vi "GOOP_VI_Item_OnPopupMenu.vi"(11 "Object":u64) -> ()   [LabVIEW 2012]
uses:
  <resource>/Framework/Providers/API/mxLvMenuItem.ctl
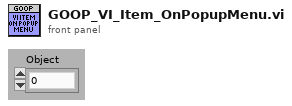
[diagram p1: front panel]
types:
  T1 = typedef "mxLvMenuItem.ctl" = cluster{"Menu Name":string, "Description":string, "Icon File Name":path, "Menu Tag":string, "Enabled":bool, "Checked":bool, "Separator":bool, "Batchable":bool, "Weight":i32, "Batch Mode (Ignored if Not Batchable)":enum32{"Show If All Items Support Command", "Show If Any Items Support Command"}, "Menu Location":enum32{"<None>", "Project", "Project / Build Specifications", "Tools", "Tools / Source Control", "Tools / Real-Time Module", "Help"}, "Exclude From Getting Started Window Menu":bool}
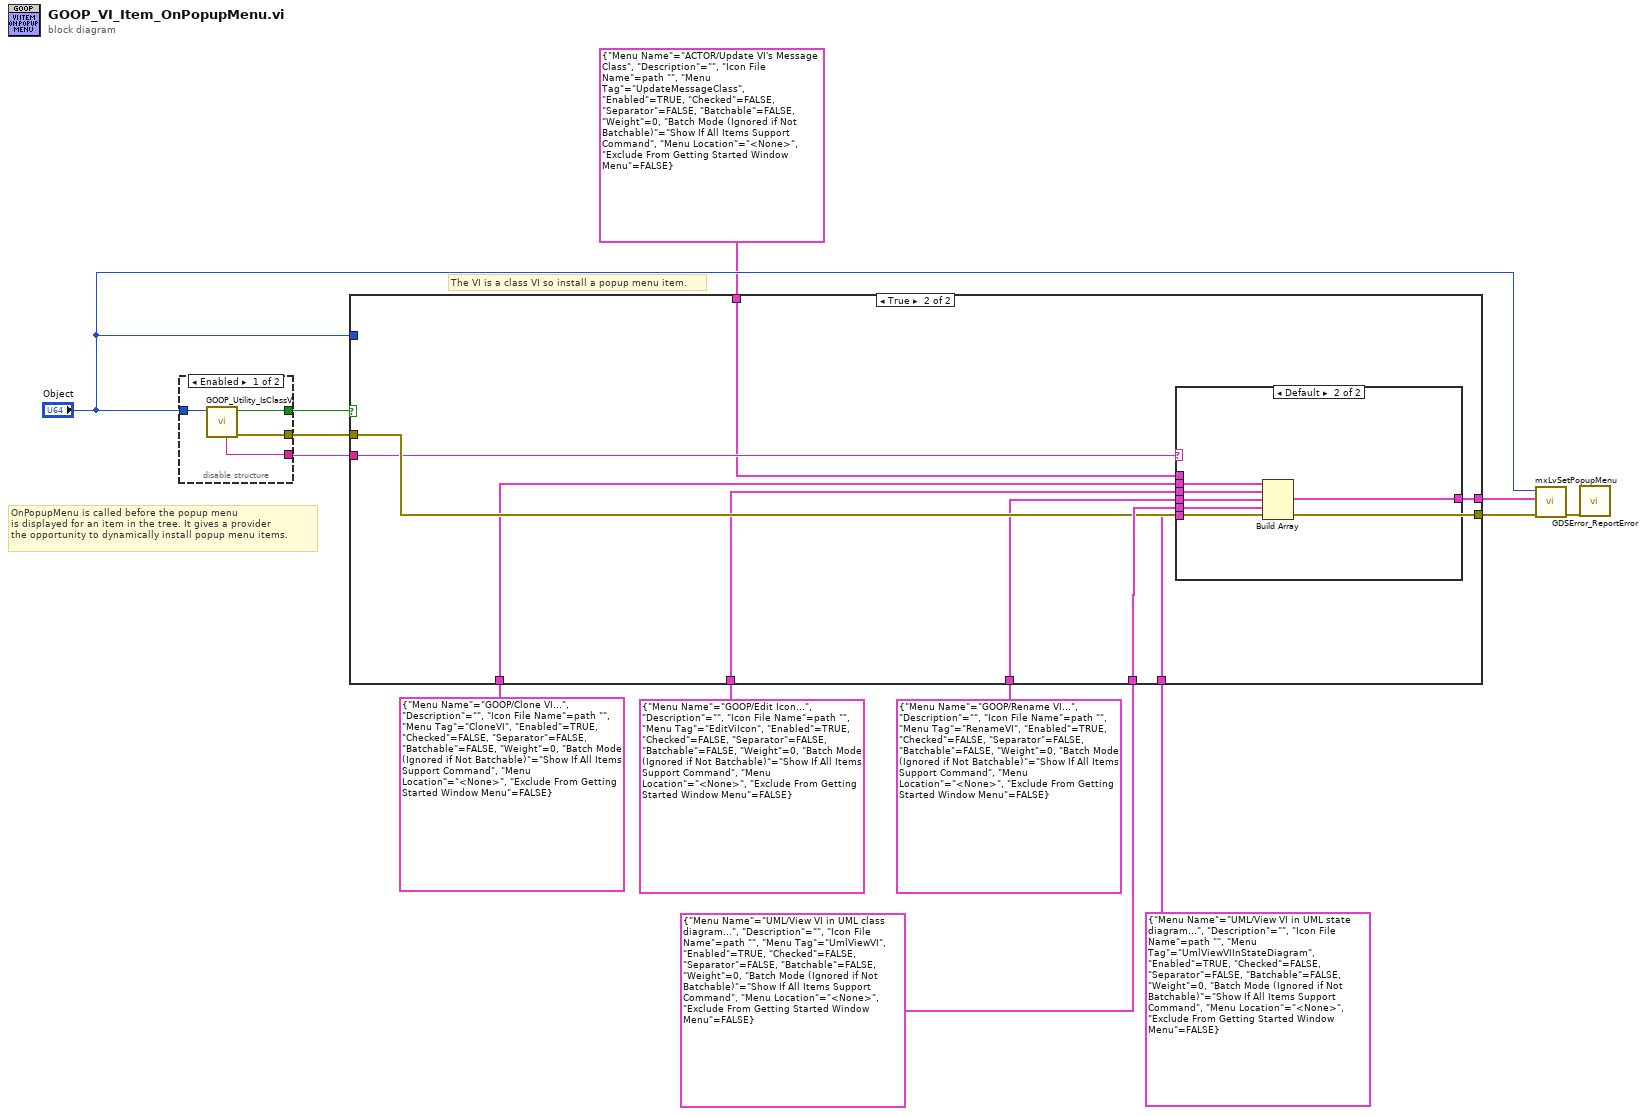
[diagram p0: block diagram]
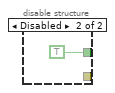
[diagram p2: hidden frame]
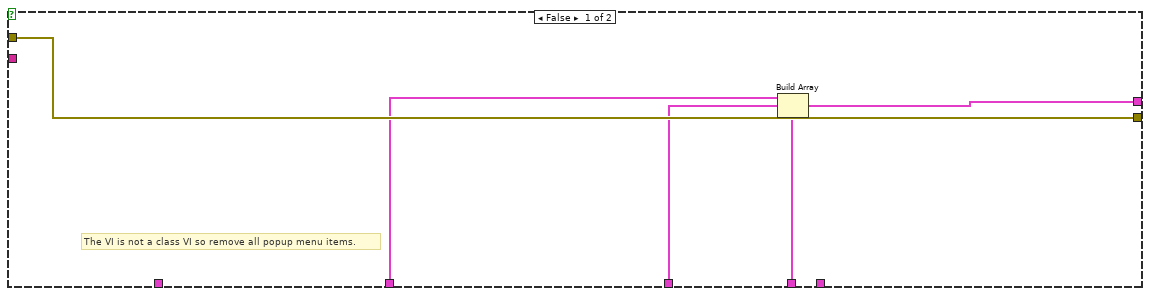
[diagram p3: hidden frame]
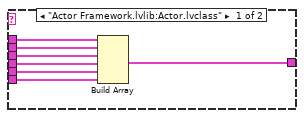
[diagram p4: hidden frame]
diagram:
  # "The VI is a class VI so install a popup menu item."
  # "OnPopupMenu is called before the popup menu\nis displayed for an item in the tree. It gives a provider\nthe opportunity to dynamically install popup menu items."
  n1 = disable-structure shown="Enabled" {
    disable-tunnel: "Object" -> [w17 _]
    disable-tunnel: [w16 _] -> w11
    disable-tunnel: [w15 TRUE ("Is Class VI?")] -> w8
    disable-tunnel: [w14 _] -> w3
    frame Enabled {
      n2 = call <resource>:"GOOP_Utility_IsClassVI.vi"("Object"=w17) -> ("error out"=w16:errorcluster, "Is Class VI?"=w15:bool, "RootClassQualified Class Name"=w14:string)  [unwired: 6 in, 2 out]
    }
    frame Disabled {
    }
  }
  n3 = case shown="True" w8 {
    tunnel: [w21 w30] -> w13
    tunnel: "Object" -> [_ _]
    tunnel: w11 -> [w23 w31]
    tunnel: T1 {"Menu Name"="UML/View VI in UML class diagram...", "Description"="", "Icon File Name"=path "", "Menu Tag"="UmlViewVI", "Enabled"=TRUE, "Checked"=FALSE, "Separator"=FALSE, "Batchable"=FALSE, "Weight"=0, "Batch Mode (Ignored if Not Batchable)"=enum."Show If All Items Support Command", "Menu Location"=enum."<None>", "Exclude From Getting Started Window Menu"=FALSE} ("Menu Item") -> [w20 w32]
    tunnel: T1 {"Menu Name"="GOOP/Clone VI...", "Description"="", "Icon File Name"=path "", "Menu Tag"="CloneVI", "Enabled"=TRUE, "Checked"=FALSE, "Separator"=FALSE, "Batchable"=FALSE, "Weight"=0, "Batch Mode (Ignored if Not Batchable)"=enum."Show If All Items Support Command", "Menu Location"=enum."<None>", "Exclude From Getting Started Window Menu"=FALSE} ("Menu Item") -> [_ w29]
    tunnel: [w23 w31] -> w7
    tunnel: T1 {"Menu Name"="GOOP/Edit Icon...", "Description"="", "Icon File Name"=path "", "Menu Tag"="EditViIcon", "Enabled"=TRUE, "Checked"=FALSE, "Separator"=FALSE, "Batchable"=FALSE, "Weight"=0, "Batch Mode (Ignored if Not Batchable)"=enum."Show If All Items Support Command", "Menu Location"=enum."<None>", "Exclude From Getting Started Window Menu"=FALSE} ("Menu Item") -> [w22 w28]
    tunnel: T1 {"Menu Name"="UML/View VI in UML state diagram...", "Description"="", "Icon File Name"=path "", "Menu Tag"="UmlViewVIInStateDiagram", "Enabled"=TRUE, "Checked"=FALSE, "Separator"=FALSE, "Batchable"=FALSE, "Weight"=0, "Batch Mode (Ignored if Not Batchable)"=enum."Show If All Items Support Command", "Menu Location"=enum."<None>", "Exclude From Getting Started Window Menu"=FALSE} ("Menu Item") -> [_ w27]
    tunnel: w3 -> [_ w26]
    tunnel: T1 {"Menu Name"="ACTOR/Update VI's Message Class", "Description"="", "Icon File Name"=path "", "Menu Tag"="UpdateMessageClass", "Enabled"=TRUE, "Checked"=FALSE, "Separator"=FALSE, "Batchable"=FALSE, "Weight"=0, "Batch Mode (Ignored if Not Batchable)"=enum."Show If All Items Support Command", "Menu Location"=enum."<None>", "Exclude From Getting Started Window Menu"=FALSE} ("Menu Item") -> [_ w25]
    tunnel: T1 {"Menu Name"="GOOP/Rename VI...", "Description"="", "Icon File Name"=path "", "Menu Tag"="RenameVI", "Enabled"=TRUE, "Checked"=FALSE, "Separator"=FALSE, "Batchable"=FALSE, "Weight"=0, "Batch Mode (Ignored if Not Batchable)"=enum."Show If All Items Support Command", "Menu Location"=enum."<None>", "Exclude From Getting Started Window Menu"=FALSE} ("Menu Item") -> [w19 w24]
    frame False {
      # "The VI is not a class VI so remove all popup menu items."
      n4 = Build Array(w22, w19, w20) -> (w21:T1[])
    }
    frame True {
      n5 = case shown="Default" w26 {
        tunnel: w32 -> [w39 w45]
        tunnel: [w38 w44] -> w30
        tunnel: w29 -> [w37 w43]
        tunnel: w28 -> [w36 w42]
        tunnel: w27 -> [w35 w41]
        tunnel: w25 -> [w34 _]
        tunnel: w24 -> [w33 w40]
        frame "Actor Framework.lvlib:Actor.lvclass" {
          n6 = Build Array(w34, w37, w36, w33, w39, w35) -> (w38:T1[])
        }
        frame Default {
          n7 = Build Array(w43, w42, w40, w45, w41) -> (w44:T1[])
        }
      }
    }
  }
  n8 = call <resource>:"mxLvSetPopupMenu.vi"("error in"=w7, "Popup Menu Items"=w13, "Item"="Object") -> ("error out"=w6:errorcluster)  [unwired: 7 in, 1 out]
  n9 = call <resource>:"GDSError_ReportError.vi"("error in (no error)"=w6) -> ()  [unwired: 18 in, 1 out]
